vi "TrafficLightSimulator.vi"() -> ()   [LabVIEW 2021]
uses:
  TrafficLightState.ctl
  CarState.ctl
panel:
  in  "Stop":bool
  out "Boolean 20":bool
  out "Boolean 19":bool
  out "Boolean 18":bool
  out "Boolean 17":bool
  out "Boolean 16":bool
  out "Boolean 15":bool
  out "Boolean 14":bool
  out "Boolean 13":bool
  out "Boolean 12":bool
  out "Boolean 11":bool
  out "Boolean 10":bool
  out "Boolean 9":bool
  out "Boolean 8":bool
  out "Boolean 7":bool
  out "Boolean 6":bool
  in  "Car Speed":dbl(knob) scale=1.0..6.0
  out "Boolean":bool
  out "Boolean 4":bool
  out "Boolean 3":bool
  out "Boolean 2":bool
  out "Boolean 5":bool
  out "HRed 2":bool
  out "Hyellow 2":bool
  out "Hgreen 2":bool
  out "VRed 2":bool
  out "Vyellow 2":bool
  out "Vgreen 2":bool
  in  "Emergency":bool
  in  "Green light (second)":dbl(knob) scale=5.0..30.0
  out "HRed":bool
  out "Hyellow":bool
  out "Hgreen":bool
  out "VRed":bool
  out "Vyellow":bool
  out "Vgreen":bool
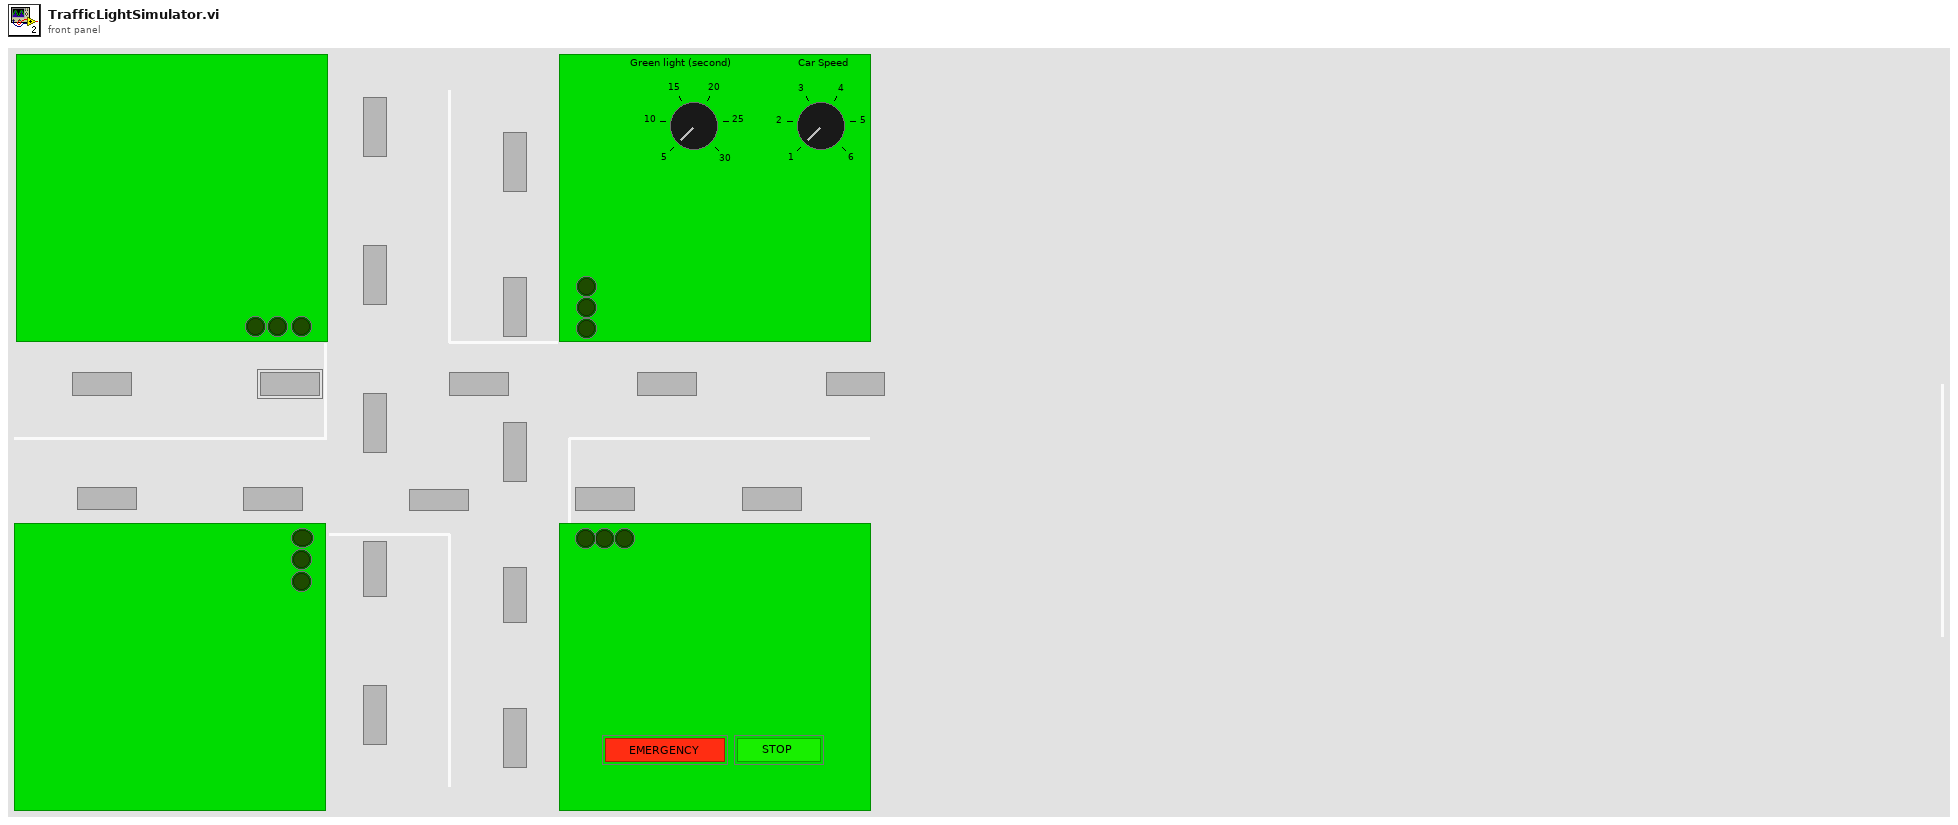
[diagram p1: front panel]
types:
  T1 = typedef "TrafficLightState.ctl" = enum16{"H1", "H2", "H3", "H4", "H5", "H6", "H7", "H8", "H9", "H10", "H11", "H12", "H13", "H14", "H15", "H16", "H17", "H18", "H19", "H20", "H21", "H22", "H23", "H24", "H25", "H26", "H27", "H28", "H29", "H30", "yellow1", "V1", "V2", "V3", "V4", "V5", "V6", "V7", "V8", "V9", "V10", "V11", "V12", "V13", "V14", "V15", "V16", "V17", "V18", "V19", "V20", "V21", "V22", "V23", "V24", "V25", "V26", "V27", "V28", "V29", "V30", "yellow2"}
  T2 = enum16{"H1", "H2", "H3", "H4", "H5", "H6", "H7", "H8", "H9", "H10", "H11", "H12", "H13", "H14", "H15", "H16", "H17", "H18", "H19", "H20", "H21", "H22", "H23", "H24", "H25", "H26", "H27", "H28", "H29", "H30", "yellow1", "V1", "V2", "V3", "V4", "V5", "V6", "V7", "V8", "V9", "V10", "V11", "V12", "V13", "V14", "V15", "V16", "V17", "V18", "V19", "V20", "V21", "V22", "V23", "V24", "V25", "V26", "V27", "V28", "V29", "V30", "yellow2"}
  T3 = typedef "CarState.ctl" = enum16{"1", "2", "3", "4", "5"}
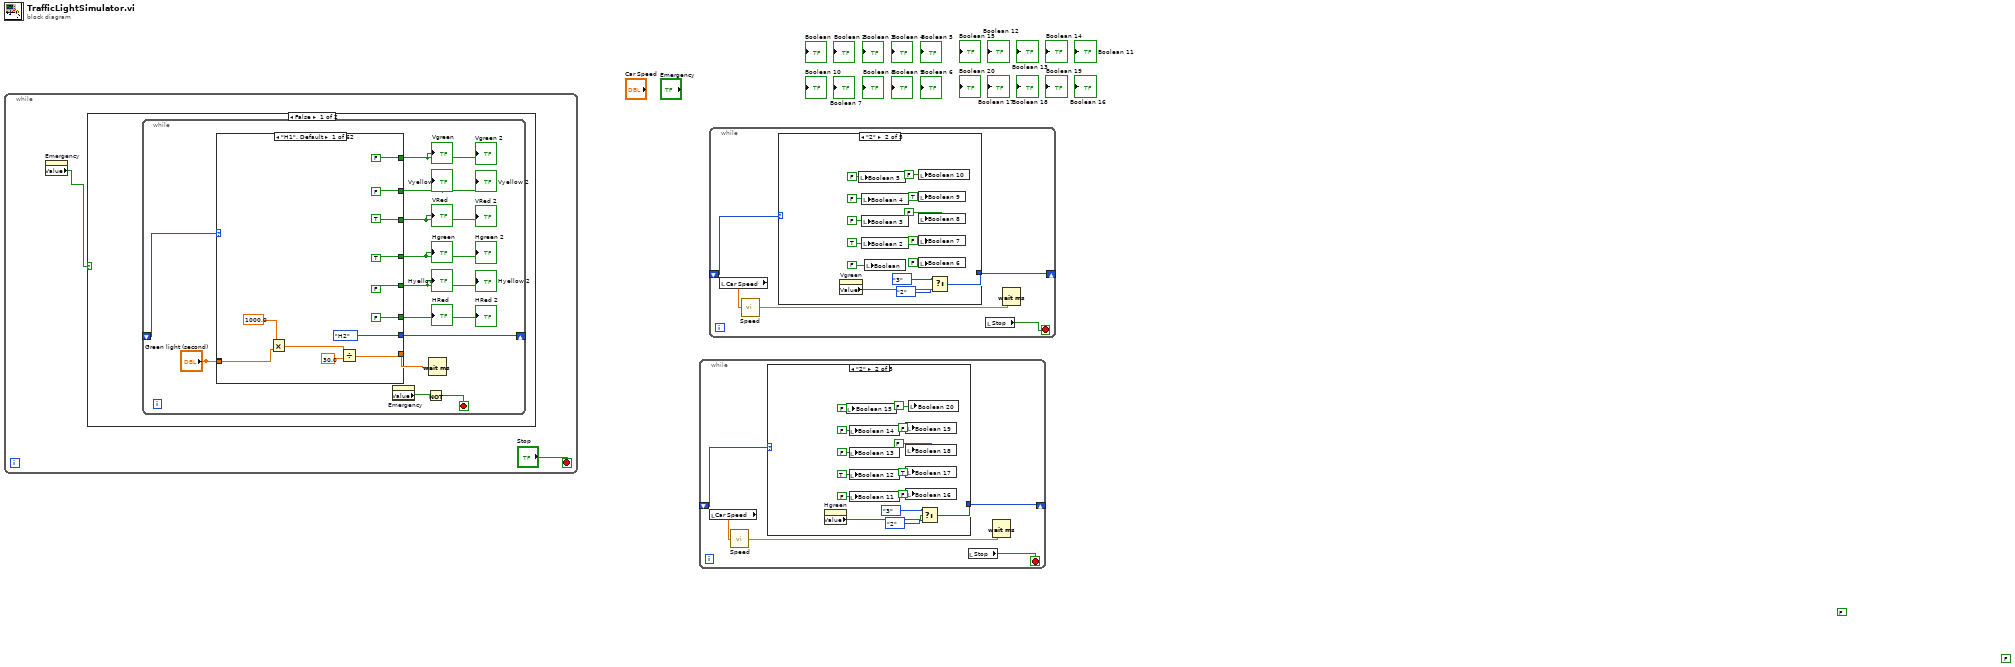
[diagram p0: block diagram]
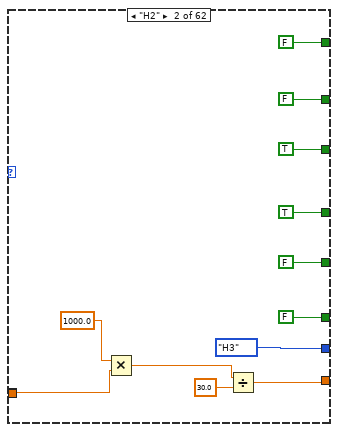
[diagram p2: hidden frame]
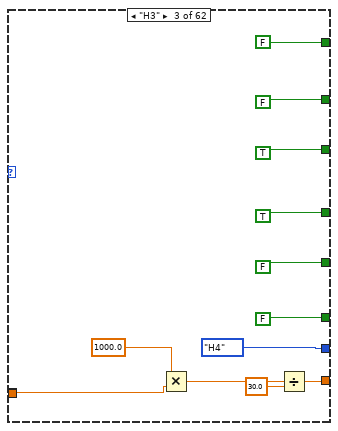
[diagram p3: hidden frame]
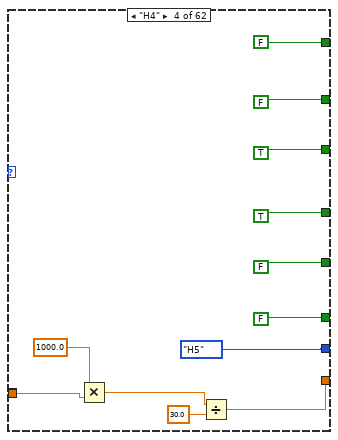
[diagram p4: hidden frame]
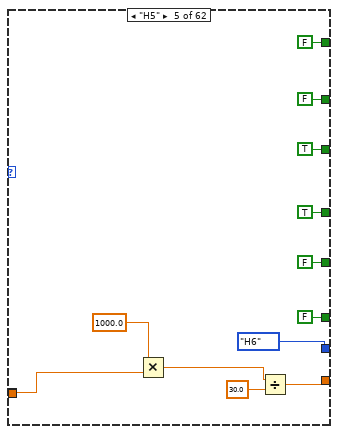
[diagram p5: hidden frame]
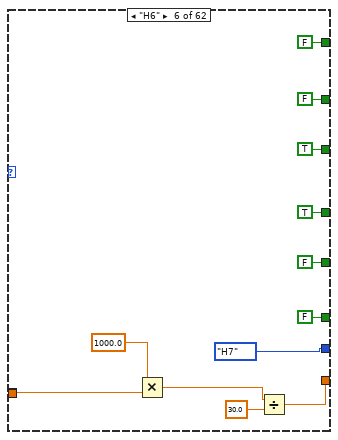
[diagram p6: hidden frame]
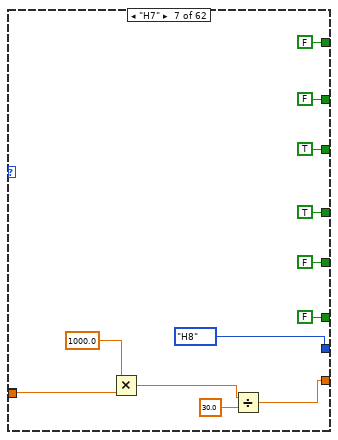
[diagram p7: hidden frame]
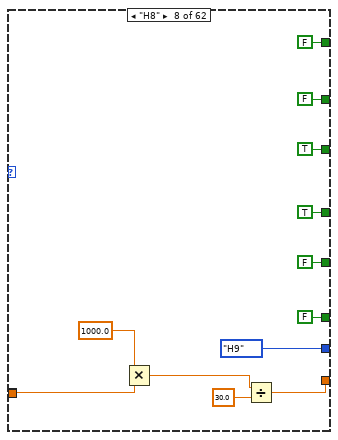
[diagram p8: hidden frame]
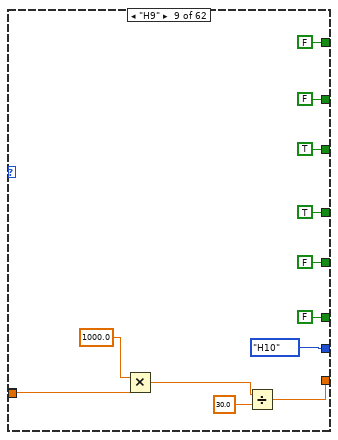
[diagram p9: hidden frame]
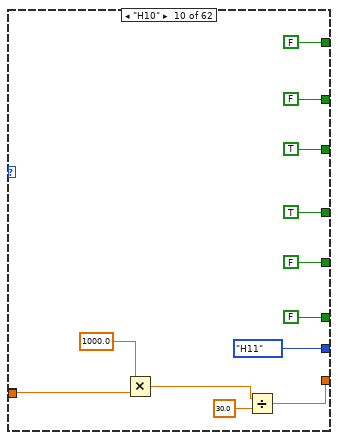
[diagram p10: hidden frame]
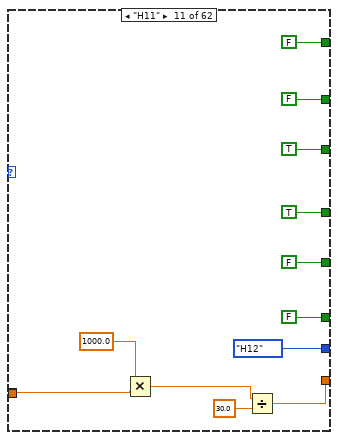
[diagram p11: hidden frame]
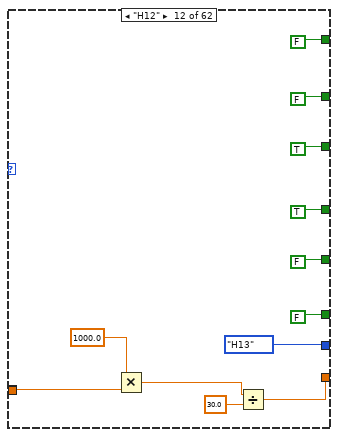
[diagram p12: hidden frame]
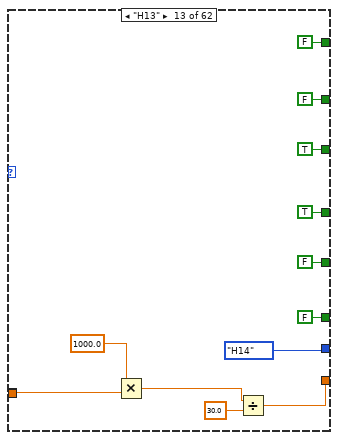
[diagram p13: hidden frame]
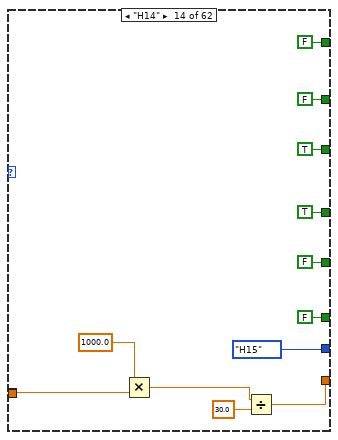
[diagram p14: hidden frame]
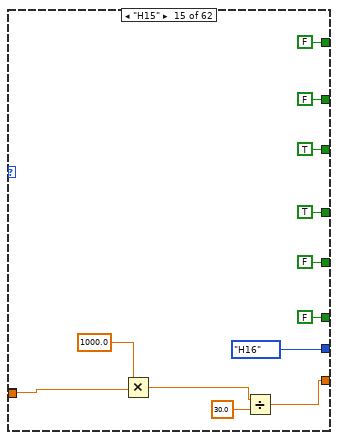
[diagram p15: hidden frame]
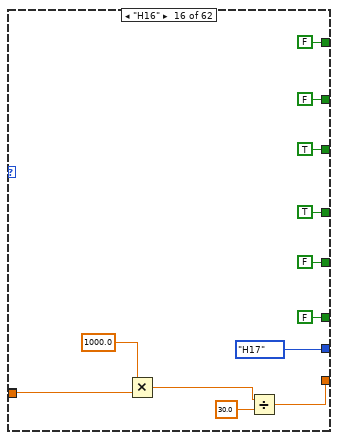
[diagram p16: hidden frame]
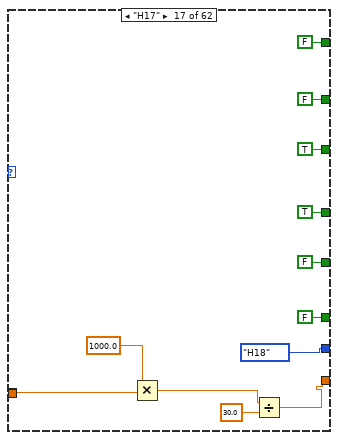
[diagram p17: hidden frame]
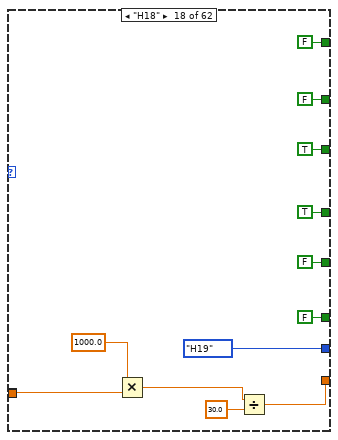
[diagram p18: hidden frame]
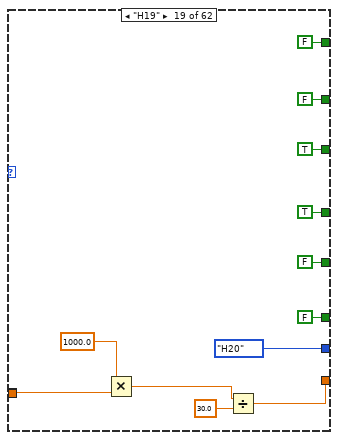
[diagram p19: hidden frame]
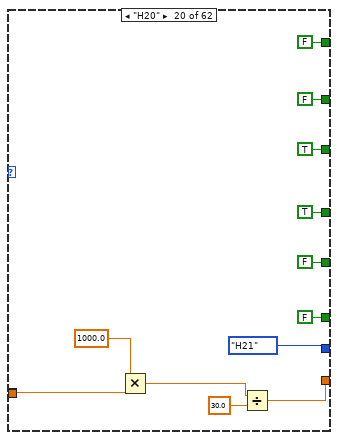
[diagram p20: hidden frame]
diagram:
  (unwired) FALSE
  (unwired) FALSE
  n1 = while {
    stop <- "Stop" stop-if-true
    n2 = property on="Emergency" class="Bool (strict)"() -> ("Value"=w2:bool)  [unwired: 2 in, 2 out]
    n3 = case shown="False" w2 {
      frame False {
        n4 = while {
          shift-right: [w5] -> _
          shift-left: _ -> [w3]
          stop <- w7 stop-if-true
          n5 = case shown="\"H1\", Default" w3 {
            tunnel: [FALSE FALSE FALSE FALSE FALSE FALSE FALSE FALSE FALSE FALSE FALSE FALSE FALSE FALSE FALSE FALSE FALSE FALSE FALSE FALSE FALSE FALSE FALSE FALSE FALSE FALSE FALSE FALSE FALSE FALSE FALSE FALSE FALSE FALSE FALSE FALSE FALSE FALSE FALSE FALSE FALSE FALSE FALSE FALSE FALSE FALSE FALSE FALSE FALSE FALSE FALSE FALSE FALSE FALSE FALSE FALSE FALSE FALSE FALSE FALSE FALSE TRUE] -> w13
            tunnel: [TRUE TRUE TRUE TRUE TRUE TRUE TRUE TRUE TRUE TRUE TRUE TRUE TRUE TRUE TRUE TRUE TRUE TRUE TRUE TRUE TRUE TRUE TRUE TRUE TRUE TRUE TRUE TRUE TRUE TRUE TRUE FALSE FALSE FALSE FALSE FALSE FALSE FALSE FALSE FALSE FALSE FALSE FALSE FALSE FALSE FALSE FALSE FALSE FALSE FALSE FALSE FALSE FALSE FALSE FALSE FALSE FALSE FALSE FALSE FALSE FALSE FALSE] -> w12
            tunnel: [FALSE FALSE FALSE FALSE FALSE FALSE FALSE FALSE FALSE FALSE FALSE FALSE FALSE FALSE FALSE FALSE FALSE FALSE FALSE FALSE FALSE FALSE FALSE FALSE FALSE FALSE FALSE FALSE FALSE FALSE TRUE FALSE FALSE FALSE FALSE FALSE FALSE FALSE FALSE FALSE FALSE FALSE FALSE FALSE FALSE FALSE FALSE FALSE FALSE FALSE FALSE FALSE FALSE FALSE FALSE FALSE FALSE FALSE FALSE FALSE FALSE FALSE] -> w10
            tunnel: [FALSE FALSE FALSE FALSE FALSE FALSE FALSE FALSE FALSE FALSE FALSE FALSE FALSE FALSE FALSE FALSE FALSE FALSE FALSE FALSE FALSE FALSE FALSE FALSE FALSE FALSE FALSE FALSE FALSE FALSE FALSE TRUE TRUE TRUE TRUE TRUE TRUE TRUE TRUE TRUE TRUE TRUE TRUE TRUE TRUE TRUE TRUE TRUE TRUE TRUE TRUE TRUE TRUE TRUE TRUE TRUE TRUE TRUE TRUE TRUE TRUE TRUE] -> w9
            tunnel: [w17 w28 w40 w53 w64 w77 w88 w100 w113 w131 w143 w154 w167 w179 w190 w203 w215 w227 w239 w250 w263 w274 w286 w298 w310 w322 w334 w347 w359 w371 1000.0 w391 w403 w415 w427 w439 w451 w462 w474 w487 w499 w511 w523 w534 w546 w558 w570 w582 w595 w607 w618 w630 w643 w655 w666 w679 w690 w702 w715 w726 w739 1000.0] -> w14
            tunnel: [TRUE TRUE TRUE TRUE TRUE TRUE TRUE TRUE TRUE TRUE TRUE TRUE TRUE TRUE TRUE TRUE TRUE TRUE TRUE TRUE TRUE TRUE TRUE TRUE TRUE TRUE TRUE TRUE TRUE TRUE FALSE FALSE FALSE FALSE FALSE FALSE FALSE FALSE FALSE FALSE FALSE FALSE FALSE FALSE FALSE FALSE FALSE FALSE FALSE FALSE FALSE FALSE FALSE FALSE FALSE FALSE FALSE FALSE FALSE FALSE FALSE FALSE] -> w11
            tunnel: "Green light (second)" -> [w19 w29 w43 _ w65 w76 w89 w101 w112 w130 w142 w155 w166 w178 w191 w202 w214 w226 w238 w251 w262 w275 w287 w299 w311 w323 w335 w346 w358 w370 _ w390 w402 _ w426 w438 w450 w463 w475 w486 w498 w510 w522 w535 w547 _ w571 w583 w594 w606 w619 w631 w642 w654 w667 w678 w691 w703 w714 w727 w738 _]
            tunnel: "Green light (second)" -> [_ _ _ w52 _ _ _ _ _ _ _ _ _ _ _ _ _ _ _ _ _ _ _ _ _ _ _ _ _ _ _ _ _ w414 _ _ _ _ _ _ _ _ _ _ _ w559 _ _ _ _ _ _ _ _ _ _ _ _ _ _ _ _]
            tunnel: [TrafficLightState."H2" ("Enum 2") TrafficLightState."H3" ("Enum 2") TrafficLightState."H4" ("Enum 2") TrafficLightState."H5" ("Enum 2") TrafficLightState."H6" ("Enum 2") T2."H7" ("Enum 2") T2."H8" ("Enum 2") T2."H9" ("Enum 2") T2."H10" ("Enum 2") T2."H11" ("Enum 2") T2."H12" ("Enum 2") T2."H13" ("Enum 2") T2."H14" ("Enum 2") T2."H15" ("Enum 2") T2."H16" ("Enum 2") T2."H17" ("Enum 2") T2."H18" ("Enum 2") T2."H19" ("Enum 2") T2."H20" ("Enum 2") T2."H21" ("Enum 2") T2."H22" ("Enum 2") T2."H23" ("Enum 2") T2."H24" ("Enum 2") T2."H25" ("Enum 2") T2."H26" ("Enum 2") T2."H27" ("Enum 2") T2."H28" ("Enum 2") T2."H29" ("Enum 2") T2."H30" ("Enum 2") T2."yellow1" ("Enum 2") T2."V1" ("Enum 2") T2."V2" ("Enum 2") T2."V3" ("Enum 2") T2."V4" ("Enum 2") T2."V5" ("Enum 2") T2."V6" ("Enum 2") TrafficLightState."V7" ("Enum 2") TrafficLightState."V8" ("Enum 2") TrafficLightState."V9" ("Enum 2") TrafficLightState."V10" ("Enum 2") TrafficLightState."V11" ("Enum 2") TrafficLightState."V12" ("Enum 2") TrafficLightState."V13" ("Enum 2") TrafficLightState."V14" ("Enum 2") TrafficLightState."V15" ("Enum 2") TrafficLightState."V16" ("Enum 2") TrafficLightState."V17" ("Enum 2") TrafficLightState."V18" ("Enum 2") TrafficLightState."V19" ("Enum 2") TrafficLightState."V20" ("Enum 2") TrafficLightState."V21" ("Enum 2") TrafficLightState."V22" ("Enum 2") TrafficLightState."V23" ("Enum 2") TrafficLightState."V24" ("Enum 2") TrafficLightState."V25" ("Enum 2") TrafficLightState."V26" ("Enum 2") TrafficLightState."V27" ("Enum 2") TrafficLightState."V28" ("Enum 2") TrafficLightState."V29" ("Enum 2") TrafficLightState."V30" ("Enum 2") TrafficLightState."yellow2" ("Enum 2") TrafficLightState."H1" ("Enum 2")] -> w5
            tunnel: [FALSE FALSE FALSE FALSE FALSE FALSE FALSE FALSE FALSE FALSE FALSE FALSE FALSE FALSE FALSE FALSE FALSE FALSE FALSE FALSE FALSE FALSE FALSE FALSE FALSE FALSE FALSE FALSE FALSE FALSE FALSE TRUE TRUE TRUE TRUE TRUE TRUE TRUE TRUE TRUE TRUE TRUE TRUE TRUE TRUE TRUE TRUE TRUE TRUE TRUE TRUE TRUE TRUE TRUE TRUE TRUE TRUE TRUE TRUE TRUE TRUE FALSE] -> w4
            frame "H1", Default {
              n6 = Multiply(x=1000.0, y=w19) -> (x*y=w18:dbl)
              n7 = Divide(x=w18, y=30.0) -> (x/y=w17:dbl)
            }
            frame "H2" {
              n8 = Multiply(x=1000.0, y=w29) -> (x*y=w32:dbl)
              n9 = Divide(x=w32, y=30.0) -> (x/y=w28:dbl)
            }
            frame "H3" {
              n10 = Multiply(x=1000.0, y=w43) -> (x*y=w41:dbl)
              n11 = Divide(x=w41, y=30.0) -> (x/y=w40:dbl)
            }
            frame "H4" {
              n12 = Multiply(x=1000.0, y=w52) -> (x*y=w55:dbl)
              n13 = Divide(x=w55, y=30.0) -> (x/y=w53:dbl)
            }
            frame "H5" {
              n14 = Multiply(x=1000.0, y=w65) -> (x*y=w67:dbl)
              n15 = Divide(x=w67, y=30.0) -> (x/y=w64:dbl)
            }
            frame "H6" {
              n16 = Multiply(x=1000.0, y=w76) -> (x*y=w79:dbl)
              n17 = Divide(x=w79, y=30.0) -> (x/y=w77:dbl)
            }
            frame "H7" {
              n18 = Multiply(x=1000.0, y=w89) -> (x*y=w91:dbl)
              n19 = Divide(x=w91, y=30.0) -> (x/y=w88:dbl)
            }
            frame "H8" {
              n20 = Multiply(x=1000.0, y=w101) -> (x*y=w103:dbl)
              n21 = Divide(x=w103, y=30.0) -> (x/y=w100:dbl)
            }
            frame "H9" {
              n22 = Multiply(x=1000.0, y=w112) -> (x*y=w116:dbl)
              n23 = Divide(x=w116, y=30.0) -> (x/y=w113:dbl)
            }
            frame "H10" {
              n24 = Multiply(x=1000.0, y=w130) -> (x*y=w133:dbl)
              n25 = Divide(x=w133, y=30.0) -> (x/y=w131:dbl)
            }
            frame "H11" {
              n26 = Multiply(x=1000.0, y=w142) -> (x*y=w145:dbl)
              n27 = Divide(x=w145, y=30.0) -> (x/y=w143:dbl)
            }
            frame "H12" {
              n28 = Multiply(x=1000.0, y=w155) -> (x*y=w157:dbl)
              n29 = Divide(x=w157, y=30.0) -> (x/y=w154:dbl)
            }
            frame "H13" {
              n30 = Multiply(x=1000.0, y=w166) -> (x*y=w169:dbl)
              n31 = Divide(x=w169, y=30.0) -> (x/y=w167:dbl)
            }
            frame "H14" {
              n32 = Multiply(x=1000.0, y=w178) -> (x*y=w181:dbl)
              n33 = Divide(x=w181, y=30.0) -> (x/y=w179:dbl)
            }
            frame "H15" {
              n34 = Multiply(x=1000.0, y=w191) -> (x*y=w193:dbl)
              n35 = Divide(x=w193, y=30.0) -> (x/y=w190:dbl)
            }
            frame "H16" {
              n36 = Multiply(x=1000.0, y=w202) -> (x*y=w205:dbl)
              n37 = Divide(x=w205, y=30.0) -> (x/y=w203:dbl)
            }
            frame "H17" {
              n38 = Multiply(x=1000.0, y=w214) -> (x*y=w217:dbl)
              n39 = Divide(x=w217, y=30.0) -> (x/y=w215:dbl)
            }
            frame "H18" {
              n40 = Multiply(x=1000.0, y=w226) -> (x*y=w229:dbl)
              n41 = Divide(x=w229, y=30.0) -> (x/y=w227:dbl)
            }
            frame "H19" {
              n42 = Multiply(x=1000.0, y=w238) -> (x*y=w241:dbl)
              n43 = Divide(x=w241, y=30.0) -> (x/y=w239:dbl)
            }
            frame "H20" {
              n44 = Multiply(x=1000.0, y=w251) -> (x*y=w253:dbl)
              n45 = Divide(x=w253, y=30.0) -> (x/y=w250:dbl)
            }
            frame "H21" {
              n46 = Multiply(x=1000.0, y=w262) -> (x*y=w265:dbl)
              n47 = Divide(x=w265, y=30.0) -> (x/y=w263:dbl)
            }
            frame "H22" {
              n48 = Multiply(x=1000.0, y=w275) -> (x*y=w277:dbl)
              n49 = Divide(x=w277, y=30.0) -> (x/y=w274:dbl)
            }
            frame "H23" {
              n50 = Multiply(x=1000.0, y=w287) -> (x*y=w289:dbl)
              n51 = Divide(x=w289, y=30.0) -> (x/y=w286:dbl)
            }
            frame "H24" {
              n52 = Multiply(x=1000.0, y=w299) -> (x*y=w301:dbl)
              n53 = Divide(x=w301, y=30.0) -> (x/y=w298:dbl)
            }
            frame "H25" {
              n54 = Multiply(x=1000.0, y=w311) -> (x*y=w313:dbl)
              n55 = Divide(x=w313, y=30.0) -> (x/y=w310:dbl)
            }
            frame "H26" {
              n56 = Multiply(x=1000.0, y=w323) -> (x*y=w325:dbl)
              n57 = Divide(x=w325, y=30.0) -> (x/y=w322:dbl)
            }
            frame "H27" {
              n58 = Multiply(x=1000.0, y=w335) -> (x*y=w337:dbl)
              n59 = Divide(x=w337, y=30.0) -> (x/y=w334:dbl)
            }
            frame "H28" {
              n60 = Multiply(x=1000.0, y=w346) -> (x*y=w349:dbl)
              n61 = Divide(x=w349, y=30.0) -> (x/y=w347:dbl)
            }
            frame "H29" {
              n62 = Multiply(x=1000.0, y=w358) -> (x*y=w361:dbl)
              n63 = Divide(x=w361, y=30.0) -> (x/y=w359:dbl)
            }
            frame "H30" {
              n64 = Multiply(x=1000.0, y=w370) -> (x*y=w373:dbl)
              n65 = Divide(x=w373, y=30.0) -> (x/y=w371:dbl)
            }
            frame "yellow1" {
            }
            frame "V1" {
              n66 = Multiply(x=1000.0, y=w390) -> (x*y=w393:dbl)
              n67 = Divide(x=w393, y=30.0) -> (x/y=w391:dbl)
            }
            frame "V2" {
              n68 = Multiply(x=1000.0, y=w402) -> (x*y=w405:dbl)
              n69 = Divide(x=w405, y=30.0) -> (x/y=w403:dbl)
            }
            frame "V3" {
              n70 = Multiply(x=1000.0, y=w414) -> (x*y=w417:dbl)
              n71 = Divide(x=w417, y=30.0) -> (x/y=w415:dbl)
            }
            frame "V4" {
              n72 = Multiply(x=1000.0, y=w426) -> (x*y=w429:dbl)
              n73 = Divide(x=w429, y=30.0) -> (x/y=w427:dbl)
            }
            frame "V5" {
              n74 = Multiply(x=1000.0, y=w438) -> (x*y=w441:dbl)
              n75 = Divide(x=w441, y=30.0) -> (x/y=w439:dbl)
            }
            frame "V6" {
              n76 = Multiply(x=1000.0, y=w450) -> (x*y=w453:dbl)
              n77 = Divide(x=w453, y=30.0) -> (x/y=w451:dbl)
            }
            frame "V7" {
              n78 = Multiply(x=1000.0, y=w463) -> (x*y=w466:dbl)
              n79 = Divide(x=w466, y=30.0) -> (x/y=w462:dbl)
            }
            frame "V8" {
              n80 = Multiply(x=1000.0, y=w475) -> (x*y=w477:dbl)
              n81 = Divide(x=w477, y=30.0) -> (x/y=w474:dbl)
            }
            frame "V9" {
              n82 = Multiply(x=1000.0, y=w486) -> (x*y=w489:dbl)
              n83 = Divide(x=w489, y=30.0) -> (x/y=w487:dbl)
            }
            frame "V10" {
              n84 = Multiply(x=1000.0, y=w498) -> (x*y=w501:dbl)
              n85 = Divide(x=w501, y=30.0) -> (x/y=w499:dbl)
            }
            frame "V11" {
              n86 = Multiply(x=1000.0, y=w510) -> (x*y=w513:dbl)
              n87 = Divide(x=w513, y=30.0) -> (x/y=w511:dbl)
            }
            frame "V12" {
              n88 = Multiply(x=1000.0, y=w522) -> (x*y=w525:dbl)
              n89 = Divide(x=w525, y=30.0) -> (x/y=w523:dbl)
            }
            frame "V13" {
              n90 = Multiply(x=1000.0, y=w535) -> (x*y=w537:dbl)
              n91 = Divide(x=w537, y=30.0) -> (x/y=w534:dbl)
            }
            frame "V14" {
              n92 = Multiply(x=1000.0, y=w547) -> (x*y=w549:dbl)
              n93 = Divide(x=w549, y=30.0) -> (x/y=w546:dbl)
            }
            frame "V15" {
              n94 = Multiply(x=1000.0, y=w559) -> (x*y=w561:dbl)
              n95 = Divide(x=w561, y=30.0) -> (x/y=w558:dbl)
            }
            frame "V16" {
              n96 = Multiply(x=1000.0, y=w571) -> (x*y=w573:dbl)
              n97 = Divide(x=w573, y=30.0) -> (x/y=w570:dbl)
            }
            frame "V17" {
              n98 = Multiply(x=1000.0, y=w583) -> (x*y=w585:dbl)
              n99 = Divide(x=w585, y=30.0) -> (x/y=w582:dbl)
            }
            frame "V18" {
              n100 = Multiply(x=1000.0, y=w594) -> (x*y=w597:dbl)
              n101 = Divide(x=w597, y=30.0) -> (x/y=w595:dbl)
            }
            frame "V19" {
              n102 = Multiply(x=1000.0, y=w606) -> (x*y=w609:dbl)
              n103 = Divide(x=w609, y=30.0) -> (x/y=w607:dbl)
            }
            frame "V20" {
              n104 = Multiply(x=1000.0, y=w619) -> (x*y=w621:dbl)
              n105 = Divide(x=w621, y=30.0) -> (x/y=w618:dbl)
            }
            frame "V21" {
              n106 = Multiply(x=1000.0, y=w631) -> (x*y=w633:dbl)
              n107 = Divide(x=w633, y=30.0) -> (x/y=w630:dbl)
            }
            frame "V22" {
              n108 = Multiply(x=1000.0, y=w642) -> (x*y=w645:dbl)
              n109 = Divide(x=w645, y=30.0) -> (x/y=w643:dbl)
            }
            frame "V23" {
              n110 = Multiply(x=1000.0, y=w654) -> (x*y=w657:dbl)
              n111 = Divide(x=w657, y=30.0) -> (x/y=w655:dbl)
            }
            frame "V24" {
              n112 = Multiply(x=1000.0, y=w667) -> (x*y=w669:dbl)
              n113 = Divide(x=w669, y=30.0) -> (x/y=w666:dbl)
            }
            frame "V25" {
              n114 = Multiply(x=1000.0, y=w678) -> (x*y=w681:dbl)
              n115 = Divide(x=w681, y=30.0) -> (x/y=w679:dbl)
            }
            frame "V26" {
              n116 = Multiply(x=1000.0, y=w691) -> (x*y=w693:dbl)
              n117 = Divide(x=w693, y=30.0) -> (x/y=w690:dbl)
            }
            frame "V27" {
              n118 = Multiply(x=1000.0, y=w703) -> (x*y=w705:dbl)
              n119 = Divide(x=w705, y=30.0) -> (x/y=w702:dbl)
            }
            frame "V28" {
              n120 = Multiply(x=1000.0, y=w714) -> (x*y=w717:dbl)
              n121 = Divide(x=w717, y=30.0) -> (x/y=w715:dbl)
            }
            frame "V29" {
              n122 = Multiply(x=1000.0, y=w727) -> (x*y=w729:dbl)
              n123 = Divide(x=w729, y=30.0) -> (x/y=w726:dbl)
            }
            frame "V30" {
              n124 = Multiply(x=1000.0, y=w738) -> (x*y=w741:dbl)
              n125 = Divide(x=w741, y=30.0) -> (x/y=w739:dbl)
            }
            frame "yellow2" {
            }
          }
          "Vgreen" <- w4
          "Vyellow" <- w13
          "VRed" <- w12
          "Hgreen" <- w11
          "Hyellow" <- w10
          "HRed" <- w9
          "Vgreen 2" <- w4
          "Vyellow 2" <- w13
          "VRed 2" <- w12
          "Hgreen 2" <- w11
          "Hyellow 2" <- w10
          "HRed 2" <- w9
          n126 = property on="Emergency" class="Bool (strict)"() -> ("Value"=w8:bool)  [unwired: 2 in, 2 out]
          n127 = Not(x=w8) -> (.not. x?=w7:bool)
          n128 = Wait (ms)(milliseconds to wait=w14) -> ()  [unwired: 1 out]
        }
      }
      frame True {
        n129 = flat-sequence {
          tunnel: [w758] -> w751
          tunnel: w751 -> [_]
          tunnel: [w772] -> _
          frame #0 {
            n130 = local write "Vgreen 2"(FALSE ("Vgreen 2")) -> ()
            n131 = local write "Vyellow 2"(TRUE ("Vyellow 2")) -> ()
            n132 = local write "HRed 2"(FALSE ("HRed 2")) -> ()
            n133 = local write "Hyellow 2"(TRUE ("Hyellow 2")) -> ()
            n134 = local write "Hgreen 2"(FALSE ("Hgreen 2")) -> ()
            n135 = local write "VRed 2"(FALSE ("VRed 2")) -> ()
            n136 = local write "Vgreen"(FALSE ("Vgreen")) -> ()
            n137 = local write "Vyellow"(TRUE ("Vyellow")) -> ()
            n138 = local write "VRed"(FALSE ("VRed")) -> ()
            n139 = local write "Hgreen"(FALSE ("Hgreen")) -> ()
            n140 = local write "Hyellow"(TRUE ("Hyellow")) -> ()
            n141 = local write "HRed"(FALSE ("HRed")) -> ()
            n142 = Wait (ms)(milliseconds to wait=u32 500) -> (millisecond timer value=w758:u32)
          }
          frame #1 {
            w766 = FALSE ("Vgreen")
            w767 = FALSE ("Vyellow")
            w768 = FALSE ("VRed")
            w769 = FALSE ("Hgreen")
            w770 = FALSE ("Hyellow")
            w771 = FALSE ("HRed")
            n143 = local write "HRed"(w771) -> ()
            n144 = local write "Hyellow"(w770) -> ()
            n145 = local write "Hgreen"(w769) -> ()
            n146 = local write "VRed"(w768) -> ()
            n147 = local write "Vyellow"(w767) -> ()
            n148 = local write "Vgreen"(w766) -> ()
            n149 = Wait (ms)(milliseconds to wait=u32 500) -> (millisecond timer value=w772:u32)
            n150 = local write "HRed 2"(w771) -> ()
            n151 = local write "Hyellow 2"(w770) -> ()
            n152 = local write "Hgreen 2"(w769) -> ()
            n153 = local write "VRed 2"(w768) -> ()
            n154 = local write "Vyellow 2"(w767) -> ()
            n155 = local write "Vgreen 2"(w766) -> ()
          }
        }
      }
    }
  }
  n156 = while {
    shift-right: [w778] -> _
    shift-left: _ -> [w777]
    stop <- w774 stop-if-true
    n157 = local read "Car Speed"() -> (w776:dbl)
    n158 = call "Speed.vi"("Speed"=w776) -> ("x-y"=w775:dbl)
    n159 = case shown="\"2\"" w777 {
      tunnel: [CarState."2" ("Enum") w788 CarState."4" ("Enum") CarState."5" ("Enum") CarState."1" ("Enum")] -> w778
      frame "1", Default {
        w779 = FALSE ("Boolean 4")
        w780 = TRUE ("Boolean")
        n160 = local write "Boolean 11"(w780) -> ()
        n161 = local write "Boolean 12"(w779) -> ()
        n162 = local write "Boolean 13"(w779) -> ()
        n163 = local write "Boolean 14"(w779) -> ()
        n164 = local write "Boolean 15"(w779) -> ()
        n165 = local write "Boolean 16"(w780) -> ()
        n166 = local write "Boolean 17"(w779) -> ()
        n167 = local write "Boolean 18"(w779) -> ()
        n168 = local write "Boolean 19"(w779) -> ()
        n169 = local write "Boolean 20"(w779) -> ()
      }
      frame "2" {
        n170 = property on="Hgreen" class="Bool (strict)"() -> ("Value"=w782:bool)  [unwired: 2 in, 2 out]
        n171 = local write "Boolean 15"(FALSE ("Boolean")) -> ()
        n172 = local write "Boolean 14"(FALSE ("Boolean 4")) -> ()
        n173 = local write "Boolean 13"(FALSE ("Boolean 3")) -> ()
        n174 = local write "Boolean 12"(TRUE ("Boolean 2")) -> ()
        n175 = local write "Boolean 11"(FALSE ("Boolean 5")) -> ()
        n176 = local write "Boolean 19"(FALSE ("Boolean 9")) -> ()
        n177 = local write "Boolean 18"(FALSE ("Boolean 8")) -> ()
        n178 = local write "Boolean 17"(TRUE ("Boolean 7")) -> ()
        n179 = local write "Boolean 16"(FALSE ("Boolean 6")) -> ()
        n180 = local write "Boolean 20"(FALSE ("Boolean 10")) -> ()
        n181 = Select(t=CarState."3" ("Enum"), s=w782, f=CarState."2" ("Enum")) -> (s? t:f=w788:T3)
      }
      frame "3" {
        n182 = local write "Boolean 19"(FALSE ("Boolean 9")) -> ()
        n183 = local write "Boolean 18"(TRUE ("Boolean 8")) -> ()
        n184 = local write "Boolean 17"(FALSE ("Boolean 7")) -> ()
        n185 = local write "Boolean 16"(FALSE ("Boolean 6")) -> ()
        n186 = local write "Boolean 20"(FALSE ("Boolean 10")) -> ()
        n187 = local write "Boolean 15"(FALSE ("Boolean")) -> ()
        n188 = local write "Boolean 14"(FALSE ("Boolean 4")) -> ()
        n189 = local write "Boolean 13"(TRUE ("Boolean 3")) -> ()
        n190 = local write "Boolean 12"(FALSE ("Boolean 2")) -> ()
        n191 = local write "Boolean 11"(FALSE ("Boolean 5")) -> ()
      }
      frame "4" {
        n192 = local write "Boolean 19"(TRUE ("Boolean 9")) -> ()
        n193 = local write "Boolean 18"(FALSE ("Boolean 8")) -> ()
        n194 = local write "Boolean 17"(FALSE ("Boolean 7")) -> ()
        n195 = local write "Boolean 16"(FALSE ("Boolean 6")) -> ()
        n196 = local write "Boolean 20"(FALSE ("Boolean 10")) -> ()
        n197 = local write "Boolean 15"(FALSE ("Boolean")) -> ()
        n198 = local write "Boolean 14"(TRUE ("Boolean 4")) -> ()
        n199 = local write "Boolean 13"(FALSE ("Boolean 3")) -> ()
        n200 = local write "Boolean 12"(FALSE ("Boolean 2")) -> ()
        n201 = local write "Boolean 11"(FALSE ("Boolean 5")) -> ()
      }
      frame "5" {
        n202 = local write "Boolean 19"(FALSE ("Boolean 9")) -> ()
        n203 = local write "Boolean 18"(FALSE ("Boolean 8")) -> ()
        n204 = local write "Boolean 17"(FALSE ("Boolean 7")) -> ()
        n205 = local write "Boolean 16"(FALSE ("Boolean 6")) -> ()
        n206 = local write "Boolean 20"(TRUE ("Boolean 10")) -> ()
        n207 = local write "Boolean 15"(TRUE ("Boolean")) -> ()
        n208 = local write "Boolean 14"(FALSE ("Boolean 4")) -> ()
        n209 = local write "Boolean 13"(FALSE ("Boolean 3")) -> ()
        n210 = local write "Boolean 12"(FALSE ("Boolean 2")) -> ()
        n211 = local write "Boolean 11"(FALSE ("Boolean 5")) -> ()
      }
    }
    n212 = local read "Stop"() -> (w774:bool)
    n213 = Wait (ms)(milliseconds to wait=w775) -> ()  [unwired: 1 out]
  }
  n214 = while {
    shift-right: [w833] -> _
    shift-left: _ -> [w832]
    stop <- w829 stop-if-true
    n215 = local read "Car Speed"() -> (w831:dbl)
    n216 = call "Speed.vi"("Speed"=w831) -> ("x-y"=w830:dbl)
    n217 = case shown="\"2\"" w832 {
      tunnel: [CarState."2" ("Enum") w843 CarState."4" ("Enum") CarState."5" ("Enum") CarState."1" ("Enum")] -> w833
      frame "1", Default {
        w834 = FALSE ("Boolean 4")
        w835 = TRUE ("Boolean")
        n218 = local write "Boolean"(w835) -> ()
        n219 = local write "Boolean 2"(w834) -> ()
        n220 = local write "Boolean 3"(w834) -> ()
        n221 = local write "Boolean 4"(w834) -> ()
        n222 = local write "Boolean 5"(w834) -> ()
        n223 = local write "Boolean 10"(w835) -> ()
        n224 = local write "Boolean 7"(w834) -> ()
        n225 = local write "Boolean 8"(w834) -> ()
        n226 = local write "Boolean 9"(w834) -> ()
        n227 = local write "Boolean 6"(w834) -> ()
      }
      frame "2" {
        n228 = property on="Vgreen" class="Bool (strict)"() -> ("Value"=w837:bool)  [unwired: 2 in, 2 out]
        n229 = local write "Boolean 5"(FALSE ("Boolean")) -> ()
        n230 = local write "Boolean 4"(FALSE ("Boolean 4")) -> ()
        n231 = local write "Boolean 3"(FALSE ("Boolean 3")) -> ()
        n232 = local write "Boolean 2"(TRUE ("Boolean 2")) -> ()
        n233 = local write "Boolean"(FALSE ("Boolean 5")) -> ()
        n234 = local write "Boolean 10"(FALSE ("Boolean 10")) -> ()
        n235 = local write "Boolean 9"(TRUE ("Boolean 9")) -> ()
        n236 = local write "Boolean 8"(FALSE ("Boolean 8")) -> ()
        n237 = local write "Boolean 7"(FALSE ("Boolean 7")) -> ()
        n238 = local write "Boolean 6"(FALSE ("Boolean 6")) -> ()
        n239 = Select(t=CarState."3" ("Enum"), s=w837, f=CarState."2" ("Enum")) -> (s? t:f=w843:T3)
      }
      frame "3" {
        n240 = local write "Boolean 4"(FALSE ("Boolean 9")) -> ()
        n241 = local write "Boolean 3"(TRUE ("Boolean 8")) -> ()
        n242 = local write "Boolean 2"(FALSE ("Boolean 7")) -> ()
        n243 = local write "Boolean 5"(FALSE ("Boolean 10")) -> ()
        n244 = local write "Boolean"(FALSE ("Boolean 6")) -> ()
        n245 = local write "Boolean 10"(FALSE ("Boolean")) -> ()
        n246 = local write "Boolean 9"(FALSE ("Boolean 4")) -> ()
        n247 = local write "Boolean 8"(TRUE ("Boolean 3")) -> ()
        n248 = local write "Boolean 7"(FALSE ("Boolean 2")) -> ()
        n249 = local write "Boolean 6"(FALSE ("Boolean 5")) -> ()
      }
      frame "4" {
        n250 = local write "Boolean 4"(TRUE ("Boolean 9")) -> ()
        n251 = local write "Boolean 3"(FALSE ("Boolean 8")) -> ()
        n252 = local write "Boolean 2"(FALSE ("Boolean 7")) -> ()
        n253 = local write "Boolean 5"(FALSE ("Boolean 10")) -> ()
        n254 = local write "Boolean"(FALSE ("Boolean 6")) -> ()
        n255 = local write "Boolean 10"(FALSE ("Boolean")) -> ()
        n256 = local write "Boolean 9"(FALSE ("Boolean 4")) -> ()
        n257 = local write "Boolean 8"(FALSE ("Boolean 3")) -> ()
        n258 = local write "Boolean 7"(TRUE ("Boolean 2")) -> ()
        n259 = local write "Boolean 6"(FALSE ("Boolean 5")) -> ()
      }
      frame "5" {
        n260 = local write "Boolean 4"(FALSE ("Boolean 9")) -> ()
        n261 = local write "Boolean 3"(FALSE ("Boolean 8")) -> ()
        n262 = local write "Boolean 2"(FALSE ("Boolean 7")) -> ()
        n263 = local write "Boolean 5"(TRUE ("Boolean 10")) -> ()
        n264 = local write "Boolean"(FALSE ("Boolean 6")) -> ()
        n265 = local write "Boolean 10"(FALSE ("Boolean")) -> ()
        n266 = local write "Boolean 9"(FALSE ("Boolean 4")) -> ()
        n267 = local write "Boolean 8"(FALSE ("Boolean 3")) -> ()
        n268 = local write "Boolean 7"(FALSE ("Boolean 2")) -> ()
        n269 = local write "Boolean 6"(TRUE ("Boolean 5")) -> ()
      }
    }
    n270 = local read "Stop"() -> (w829:bool)
    n271 = Wait (ms)(milliseconds to wait=w830) -> ()  [unwired: 1 out]
  }
